vi "Shooter Loop.vi"   [LabVIEW 2015]
uses:
  Common Code/Shooter State.ctl
  Robot Global Data.vi
types:
  T1 = typedef "Shooter Command Cluster.ctl" = cluster{"Command":T2, "Mode":T3, "Shot Type":T4, "Override Trigger IR":bool, "Override Angle?":bool}
  T2 = typedef "Shooter Commands.ctl" = enum16{"Idle", "Prime Shooter", "Shoot"}
  T3 = typedef "Shoot Modes Enum.ctl" = enum16{"Manual", "Safe", "Auto"}
  T4 = typedef "Shot Type.ctl" = enum16{"Batter Shot", "Corner Shot", "Curve Shot", "Vision Shot", "Deep Middle Shot"}
  T5 = typedef "Manual Shoot.ctl" = cluster{"Spin Wheels":bool, "Fire":bool, "Angle":dbl, "Angle Power":dbl, "Use Manual Angle":bool, "Override RPM":bool, "Left RPM":dbl, "Right RPM":dbl, "Secure Ball?":bool}
  T6 = typedef "WPI_DigitalInputDevRef.ctl" = cluster{"DevStatus":errorcluster, "DIO Channel":T7}
  T7 = typedef "FPGA_DIOChannel.ctl" = enum8{"DIO 0", "DIO 1", "DIO 2", "DIO 3", "DIO 4", "DIO 5", "DIO 6", "DIO 7", "DIO 8", "DIO 9", "DIO MXP 0", "DIO MXP 1", "DIO MXP 2", "DIO MXP 3", "DIO MXP 4", "DIO MXP 5", "DIO MXP 6", "DIO MXP 7", "DIO MXP 8", "DIO MXP 9", "DIO MXP 10", "DIO MXP 11", "DIO MXP 12", "DIO MXP 13", "DIO MXP 14", "DIO MXP 15", "Invalid"}
  T8 = typedef "Shooter State.ctl" = enum16{"Idle", "Warmup", "Shooter Ready", "Shoot"}
  T9 = typedef "WPI_MotorControlDeviceRef.ctl" = cluster{"DeviceStatus":errorcluster, "Type":T10, "PWM":cluster{"PWM Channel":T11, "DeadBand":T12}, "CAN":cluster{"Device Number":u8, "Control Mode":T13, "Semaphore":T14, "Max Vout":dbl, "TalonSRX Control Mode":T15}, "Invert":bool}
  T10 = typedef "WPI_MotorControlType.ctl" = enum16{"PWM", "CAN", "CANTalonSRX"}
  T11 = typedef "FPGA_DIOPWMChannel.ctl" = enum8{"PWM 0", "PWM 1", "PWM 2", "PWM 3", "PWM 4", "PWM 5", "PWM 6", "PWM 7", "PWM 8", "PWM 9", "PWM MXP 0", "PWM MXP 1", "PWM MXP 2", "PWM MXP 3", "PWM MXP 4", "PWM MXP 5", "PWM MXP 6", "PWM MXP 7", "PWM MXP 8", "PWM MXP 9", "Invalid"}
  T12 = typedef "WPI_PWMDeadband.ctl" = cluster{"Name":string, "maxPositivePwm":i32, "minPositivePwm":i32, "centerPwm":i32, "maxNegativePwm":i32, "minNegativePwm":i32, "angularRange":u16}
  T13 = typedef "WPI_CANJaguar_ControlMode.ctl" = enum8{"Percent VBus", "Current", "Speed", "Position", "Voltage"}
  T14 = typedef "Semaphore RefNum" = refnum<k1>
  T15 = typedef "WPI_CANTalonSRX_APIControlMode.ctl" = enum8{"Percent VBus", "Speed", "Position", "Slave", "Unchanged / Invalid", "Voltage Compensation", "Current", "Motion Profile"}
  T16 = typedef "Dashboard Control Data.ctl" = cluster{"Shooter Presets":T17, "Encoder Control":T19, "Steer PID output":cluster{"output high":dbl, "output low":dbl}, " Steer PID gains":cluster{"proportional gain (Kc)":dbl, "integral time (Ti, min)":dbl, "derivative time (Td, min)":dbl}, "Drivetrain Settings":T20, "Vision Packet":T21, "Dashboard Drivetrain Command":T22, "Info/Command Cluster":T24, "Ball Vision Packet":T25, "Intake Presets":T27, "Intake Encoder Control":T29, "Climb Presets":T30, "Ultrasonic Limit":dbl, "Roll Limit":dbl, "Pitch Limit":dbl, "Goal Output Range":cluster{"output high":dbl, "output low":dbl}}
  T17 = typedef "Shooter Presets.ctl" = cluster{"Batter Shot":T18, "Deep Middle Shot":T18, "Manual Shot":T18, "Left Ticks Per Rotation":dbl, "Right Ticks Per Rotation":dbl, "Low Bar Shot":T18, "Shooter RPM Tolerance":dbl, "IIR Filter Power":dbl, "Trigger Power":dbl, "Fire from Load Delay":i32, "Angle Pot M":dbl, "Angle Pot B":dbl, "Shooter Length":dbl, "String Pot Dist":dbl, "Angle PID gains":cluster{"proportional gain (Kc)":dbl, "integral time (Ti, min)":dbl, "derivative time (Td, min)":dbl}, "Angle Motor Output":cluster{"output high":dbl, "output low":dbl}, "Shooter Angle Tolerance":dbl, "Vision Shoot x^2":dbl, "Vision Shoot x":dbl, "Dist from Axis Cam to Pivot":dbl, "High Goal Center Height":dbl, "Feed Forward Max Accel":dbl, "Feed Forward Kv":dbl, "Backwards Trigger":dbl, "Shot Finish Delay (ms)":dbl, "Angle Max Current":dbl, "Angle Current Trip Time":dbl, "Shooter Intake Angle":dbl, "Vision Shoot c":dbl, "Reset?":bool, "Servo Release Delay":dbl, "Servo Idle Angle":i32, "Servo Hold Angle":i32, "Angle Pot x^2":dbl, "Angle Pot x":dbl, "Angle Pot c":dbl, "Ignore Angle?":bool}
  T18 = typedef "Shot Presets.ctl" = cluster{"Left Wheel RPM":dbl, "Right Wheel RPM":dbl, "Angle":dbl}
  T19 = typedef "Encoder Control.ctl" = cluster{"Right Tick Constant":dbl, "Left Tick Constant":dbl, "Reset?":bool, "Y Dist":cluster{"PID gains":cluster{"proportional gain (Kc)":dbl, "integral time (Ti, min)":dbl, "derivative time (Td, min)":dbl}}, "Y Stop Thresh":dbl, "Y Stop Speed":dbl}
  T20 = typedef "Drivetrain Settings.ctl" = cluster{"Gyro Tolerance":dbl, "Throttle Ramp (ms)":dbl, "Angular rate compensation":bool, "Throttle to Rate Scale":dbl, "Rate compensation gain":dbl, "Kv":dbl, "Ka":dbl, "Feed Forward P":dbl, "Feed Forward D":dbl, "Goal Vision PID gains":cluster{"proportional gain (Kc)":dbl, "integral time (Ti, min)":dbl, "derivative time (Td, min)":dbl}, "Goal Detection Window":dbl}
  T21 = typedef "Goal Vision Packet.ctl" = cluster{"Distance":dbl, "Center X":dbl, "Center Y":dbl, "Found Target?":bool}
  T22 = typedef "Dashboard Drivetrain Command.ctl" = cluster{"Drivetrain Vision":T23}
  T23 = typedef "Drivetrain Vision.ctl" = cluster{"Goal Window":dbl, "Ball Window":dbl}
  T24 = typedef "Ball Tracking Command Cluster.ctl" = cluster{"Distance to Ball":dbl, "Desired Angle":dbl, "Command":enum16{"Turn to Ball", "Turn to Angle", "Get Distance"}, "Pixels from Center":dbl}
  T25 = typedef "Ball Vision Packet.ctl" = cluster{"Ball Detected?":bool, "Distance to Ball":dbl, "Desired Angle":dbl, "Pixels from Center":dbl, "Tracking mode":T26}
  T26 = typedef "Tracking Mode.ctl" = enum16{"Turn to Ball", "Turn to Angle"}
  T27 = typedef "Intake Presets.ctl" = cluster{"Intake Speed":dbl, "Outake Speed":dbl, "Low Height":dbl, "Half Height":dbl, "Full Height":dbl, "Angle Speed":dbl, "Fast Angle":dbl, "Encoder Scale":dbl, "Load Height":dbl, "Output Range":T28, "Rotation Power Max/Min":dbl, "MaxCurrent":dbl, "Intake Trip Time":dbl, "Idle Height":dbl, "Max Height":dbl, "Reset Encoders?":bool, "PID gains":cluster{"proportional gain (Kc)":dbl, "integral time (Ti, min)":dbl, "derivative time (Td, min)":dbl}}
  T28 = typedef "Drivetrain Output Range.ctl" = cluster{"output high":dbl, "output low":dbl}
  T29 = typedef "IntakeEcoderControl.ctl" = cluster{"Arm Tick Constant":dbl, "Reset?":bool, "Y Dist":cluster{"PID gains":cluster{"proportional gain (Kc)":dbl, "integral time (Ti, min)":dbl, "derivative time (Td, min)":dbl}}, "Y Stop Thresh":dbl, "Y Stop Speed":dbl}
  T30 = typedef "Climb Presets.ctl" = cluster{"Pull Power":dbl, "Unpin Power":dbl, "Time to Hold":dbl}
  T31 = typedef "Shooter State Cluster.ctl" = cluster{"State":T8, "Left RPM":dbl, "Right RPM":dbl, "Shooter Ready?":bool, "Ball Loaded?":bool, "Current Angle":dbl, "Angle Motor Output":dbl, "Trigger Output":dbl, "Angle Ready?":bool, "RPM Ready?":bool, "Vision Ready?":bool, "Ball Loaded?":bool, "Mode":T3, "Shot Type":T4, "Pot Height":dbl, "Current Tripped Forward?":bool, "Current Tripped Backward?":bool, "Left Motor":dbl, "Right Motor":dbl, "Intake High?":bool, "Raw Left Pos":dbl, "Raw Right Pos":dbl, "Raw Left V":dbl, "Raw Right V":dbl, "Right Servo":i32, "Left Servo":i32}
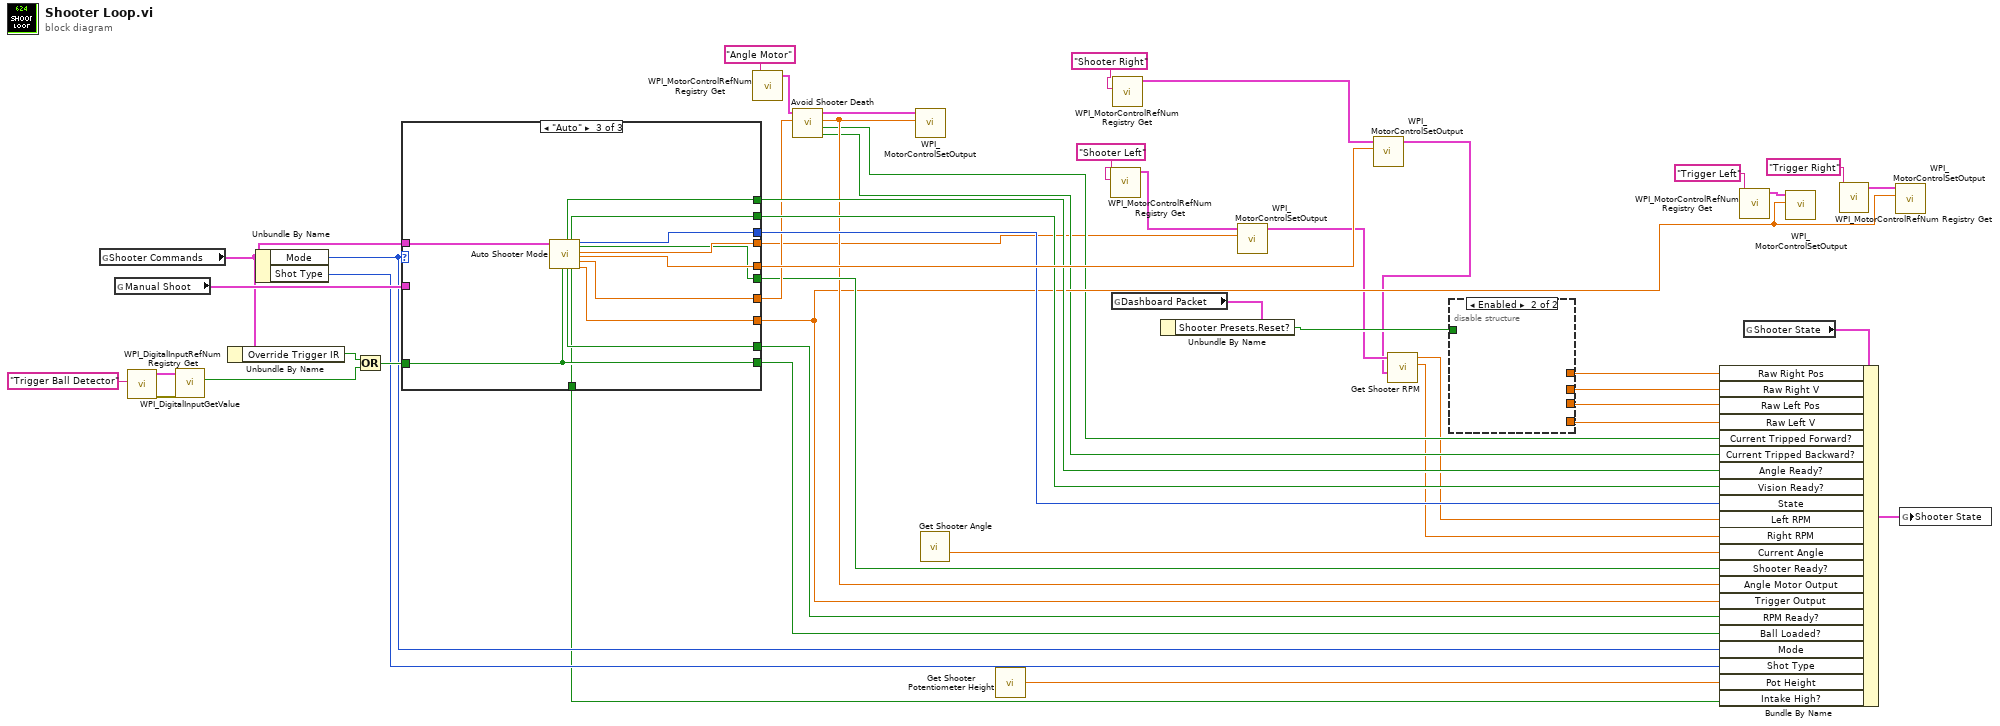
[diagram p0: block diagram]
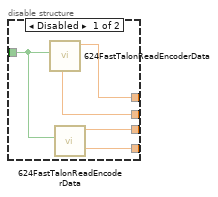
[diagram p2: hidden frame]
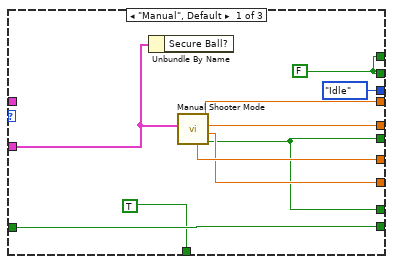
[diagram p3: hidden frame]
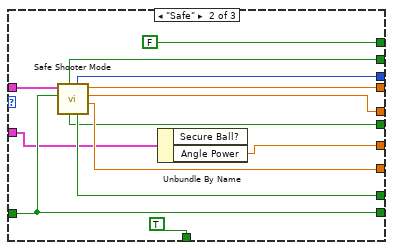
[diagram p4: hidden frame]
diagram:
  n1 = global read "Robot Global Data.vi" "Shooter Commands"() -> (w41:T1)
  n2 = global read "Robot Global Data.vi" "Manual Shoot"() -> (w47:T5)
  n3 = call <vilib>:"WPI_DigitalInputRefNum Registry Get.vi"("refnum name"="Trigger Ball Detector") -> ("error out"=w44:errorcluster, "DigitalInputDevRef"=w43:T6)  [unwired: 9 in]
  n4 = call <vilib>:"WPI_DigitalInputGetValue.vi"("error in (no error)"=w44, "DigitalInputDevRef"=w43) -> ("Value"=w39:bool)  [unwired: 7 in, 2 out]
  n5 = Unbundle By Name(w41) -> ("Override Trigger IR"=w40:bool)
  n6 = Unbundle By Name(w41) -> ("Mode"=w31:T3, "Shot Type"=w30:T4)
  n7 = Or(x=w40, y=w39) -> (x .or. y?=w38:bool)
  n8 = case shown="\"Auto\"" w31 {
    tunnel: w41 -> [_ w72 w84]
    tunnel: w47 -> [w50 w62 _]
    tunnel: [w59 w70 w78] -> w6
    tunnel: [w56 w69 w79] -> w45
    tunnel: [w54 w64 w74] -> w27
    tunnel: w38 -> [w58 w71 w83]
    tunnel: [w58 w71 w83] -> w35
    tunnel: [w57 w61 w80] -> w29
    tunnel: [w55 w68 w81] -> w17
    tunnel: [w54 w66 w82] -> w34
    tunnel: [Shooter_State."Idle" ("State") w67 w77] -> w36
    tunnel: [w52 w65 w76] -> w32
    tunnel: [w52 FALSE ("Angle In Range?") w75] -> w33
    tunnel: [TRUE ("Intake High Angle Allowed?") TRUE ("Intake High Angle Allowed?") w73] -> w22
    frame "Manual", Default {
      w52 = FALSE ("Vision Target Aligned?")
      n9 = Unbundle By Name(w50) -> ()  [unwired: 1 out]
      n10 = call "Manual Shooter Mode.vi"("Manual Shoot"=w50) -> ("Shooter Ready?"=w54:bool, "Trigger Output"=w55:dbl, "Right Output"=w56:dbl, "Left Output"=w59:dbl, "Angle Motor Out"=w57:dbl)  [unwired: 6 in]
    }
    frame "Safe" {
      n11 = call "Safe Shooter Mode.vi"("Ball Detected?"=w71, "Shooter Commands"=w72) -> ("Trigger Power"=w68:dbl, "Right Power"=w69:dbl, "Left Power"=w70:dbl, "RPM Ready?"=w66:bool, "State"=w67:T8, "Shooter Ready?"=w64:bool, "Vision Ready?"=w65:bool)  [unwired: 3 in]
      n12 = Unbundle By Name(w62) -> ("Angle Power"=w61:dbl)  [unwired: 1 out]
    }
    frame "Auto" {
      n13 = call "Auto Shooter Mode.vi"("Shooter Command"=w84, "Ball Loaded?"=w83) -> ("Angle In Range?"=w75:bool, "RPM Ready?"=w82:bool, "Vision Target Aligned?"=w76:bool, "Intake High Angle Allowed?"=w73:bool, "State"=w77:T8, "Shooter Ready?"=w74:bool, "Left Output"=w78:dbl, "Right Output"=w79:dbl, "Angle Motor Output"=w80:dbl, "Trigger Output"=w81:dbl)  [unwired: 7 in, 1 out]
    }
  }
  n14 = call <vilib>:"WPI_MotorControlRefNum Registry Get.vi"("refnum name"="Angle Motor") -> ("MotorControlDevRef"=w28:T9)  [unwired: 9 in, 1 out]
  n15 = call "Avoid Shooter Death.vi"("Proposed Power"=w29, "CAN Talon SRX Ref 3"=w28) -> ("Reverse Trip?"=w15:bool, "Forward Trip?"=w16:bool, "Actual Output"=w25:dbl, "CAN Talon SRX Ref 4"=w26:T9)  [unwired: 6 in]
  n16 = call <vilib>:"WPI_MotorControlSetOutput.vi"("Output"=w25, "MotorControlDevRef"=w26) -> ()  [unwired: 7 in, 3 out]
  n17 = call "Get Shooter Angle.vi"() -> ("Current Angle"=w24:dbl)  [unwired: 11 in]
  n18 = call "Get Shooter Potentiometer Height.vi"() -> ("Height"=w23:dbl)  [unwired: 11 in]
  n19 = call <vilib>:"WPI_MotorControlRefNum Registry Get.vi"("refnum name"="Shooter Left") -> ("MotorControlDevRef"=w2:T9)  [unwired: 9 in, 1 out]
  n20 = global read "Robot Global Data.vi" "Dashboard Packet"() -> (w8:T16)
  n21 = call <vilib>:"WPI_MotorControlRefNum Registry Get.vi"("refnum name"="Shooter Right") -> ("MotorControlDevRef"=w1:T9)  [unwired: 9 in, 1 out]
  n22 = Unbundle By Name(w8) -> ("Shooter Presets.Reset?"=w7:bool)
  n23 = call <vilib>:"WPI_MotorControlSetOutput.vi"("Output"=w6, "MotorControlDevRef"=w2) -> ("MotorControlDevRef"=w4:T9)  [unwired: 7 in, 2 out]
  n24 = call <vilib>:"WPI_MotorControlSetOutput.vi"("Output"=w45, "MotorControlDevRef"=w1) -> ("MotorControlDevRef"=w3:T9)  [unwired: 7 in, 2 out]
  n25 = call "Get Shooter RPM.vi"("Right Shooter Wheel"=w3, "Left Shooter Wheel"=w4) -> ("Right RPM"=w13:dbl, "Left RPM"=w14:dbl)  [unwired: 7 in, 1 out]
  n26 = disable-structure shown="Enabled" {
    disable-tunnel: [w90 _] -> w12
    disable-tunnel: [w89 _] -> w11
    disable-tunnel: [w88 _] -> w10
    disable-tunnel: [w87 _] -> w9
    disable-tunnel: w7 -> [w86 _]
    frame Disabled {
      n27 = call "624FastTalonReadEncoderData.vi"("Reset?"=w86) -> ("Sensor RPM"=w89:dbl, "Sensor Position"=w90:dbl)  [unwired: 9 in]
      n28 = call "624FastTalonReadEncoderData.vi"("Reset?"=w86) -> ("Sensor RPM"=w87:dbl, "Sensor Position"=w88:dbl, "CAN Talon SRX Ref"=w85:T9)  [unwired: 8 in]
    }
    frame Enabled {
    }
  }
  n29 = call <vilib>:"WPI_MotorControlRefNum Registry Get.vi"("refnum name"="Trigger Left") -> ("MotorControlDevRef"=w19:T9)  [unwired: 9 in, 1 out]
  n30 = global read "Robot Global Data.vi" "Shooter State"() -> (w49:T31)
  n31 = Bundle By Name(cluster=w49, "Raw Right Pos"=w12, "Raw Right V"=w11, "Raw Left Pos"=w10, "Raw Left V"=w9, "Current Tripped Forward?"=w16, "Current Tripped Backward?"=w15, "Angle Ready?"=w33, "Vision Ready?"=w32, "State"=w36, "Left RPM"=w14, "Right RPM"=w13, "Current Angle"=w24, "Shooter Ready?"=w27, "Angle Motor Output"=w25, "Trigger Output"=w17, "RPM Ready?"=w34, "Ball Loaded?"=w35, "Mode"=w31, "Shot Type"=w30, "Pot Height"=w23, "Intake High?"=w22) -> (w48:T31)
  n32 = call <vilib>:"WPI_MotorControlSetOutput.vi"("Output"=w17, "MotorControlDevRef"=w19) -> ()  [unwired: 7 in, 3 out]
  n33 = call <vilib>:"WPI_MotorControlRefNum Registry Get.vi"("refnum name"="Trigger Right") -> ("MotorControlDevRef"=w18:T9)  [unwired: 9 in, 1 out]
  n34 = call <vilib>:"WPI_MotorControlSetOutput.vi"("Output"=w17, "MotorControlDevRef"=w18) -> ()  [unwired: 7 in, 3 out]
  n35 = global write "Robot Global Data.vi" "Shooter State"(w48) -> ()
